vi "Init.vi"(8 "error in":errorcluster, 11 "CFG Base in":refnum<class "Red-y Pressure Control CFG.lvclass">) -> (0 "error out":errorcluster, 3 "CFG Base out":refnum<class "Red-y Pressure Control CFG.lvclass">)   [LabVIEW 2024, in "Red-y Pressure Control CFG.lvclass"]
uses:
  Red-y Pressure Control CFG.lvclass
  Red-y Pressure Control CFG.lvclass/Red-y Pressure Control CFG.ctl
  Configurations/CFG Base/CFG Base.lvclass/CFG Base.ctl
  f61d1269-8a73-4422-950f-b7b3d93ad04d.vi
  3e784602-24e4-4a87-8e8a-87b1468842a3.vi
  f61d1269-8a73-4422-950f-b7b3d93ad04d.vi/a4169a97-72fc-4003-a778-603cf20cafa0.vi
  3e784602-24e4-4a87-8e8a-87b1468842a3.vi/a4169a97-72fc-4003-a778-603cf20cafa0.vi
  <vilib>/JDP Science/JSONtext/Find Item.vi
  <vilib>/JDP Science/JSONtext/Next JSON Value.vi
  <vilib>/JDP Science/JSONtext/String Subset.vi
  <vilib>/JDP Science/JSONtext/Parsing/Advance past next JSON Value (inlined COPY).vi
  <vilib>/JDP Science/JSONtext/Parsing/Advance past whitespace.vi
  <vilib>/JDP Science/JSONtext/Parsing/Advance past String.vi
  <vilib>/JDP Science/JSONtext/Parsing/Advance past Number.vi
  <vilib>/JDP Science/JSONtext/Parsing/Advance past Line Ending.vi
  <vilib>/JDP Science/JSONtext/Parsing/Parse Full Path or Item Name.vi
  <vilib>/JDP Science/JSONtext/Parsing/Advance past Array.vi
  <vilib>/JDP Science/JSONtext/Parsing/Advance past Object.vi
  <vilib>/JDP Science/JSONtext/support/Error Cluster From Code.vi
  <vilib>/JDP Science/JSONtext/Offset/Find Item Locations by Path.vi
  <vilib>/JDP Science/JSONtext/JSON text to Variant.vi
  <vilib>/Utility/error.llb/Error Cluster From Error Code.vi
  <vilib>/JDP Science/JSONtext/LVClass Serializer/JSONtext LVClass Serializer.lvclass
  Voegtlin_NI_SMART_Modbus_Drivers/Voegtlin_NI_SMART_Modbus_Drivers.lvlib
  Configurations/CFG Base/CFG Base.lvclass
  Configurations/CFG JSON/CFG JSON.lvclass
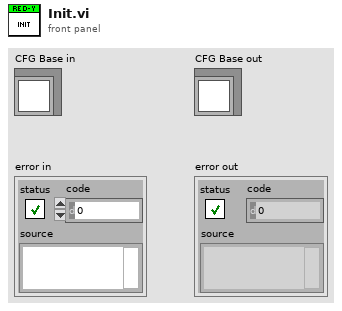
[diagram p1: front panel]
types:
  T1 = cluster{"COM Port Selected":string, "Data out":i32}
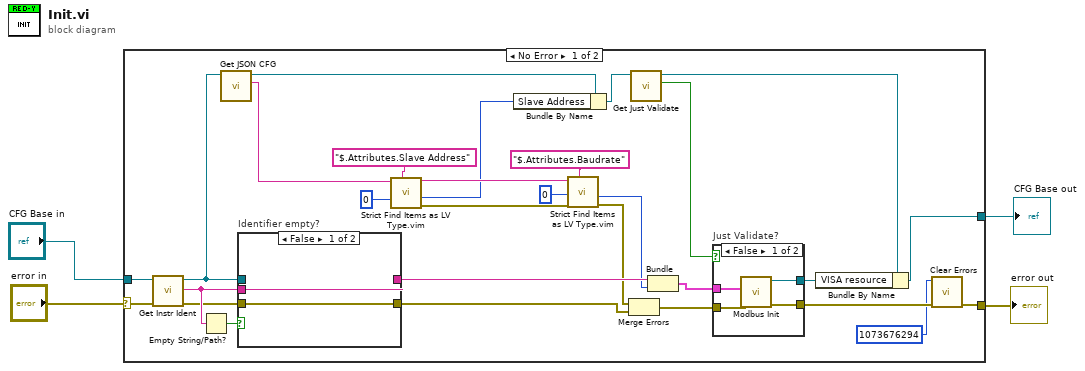
[diagram p0: block diagram]
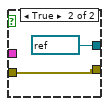
[diagram p2: hidden frame]
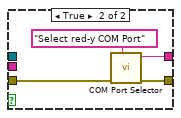
[diagram p3: hidden frame]
diagram:
  n1 = case shown="No Error" "error in" {
    selector: "error in" -> [w33 w46]
    tunnel: "CFG Base in" -> [w32 w47]
    tunnel: [w30 w47] -> w2
    tunnel: [w21 w46] -> w1
    frame No Error {
      n2 = call-dynamic "Get Instr Ident.vi"("error in"=w33, "CFG JSON in"=w32) -> ("error out"=w24:errorcluster, "Instr Ident"=w29:string, "CFG JSON out"=w25:refnum<class "Red-y Pressure Control CFG.lvclass">)  [unwired: 7 in]
      n3 = Empty String/Path?(string/path=w29) -> (empty?=w31:bool)
      n4 = call "Get JSON CFG.vi"("CFG JSON in"=w25) -> ("<JSON> CFG"=w9:string, "CFG JSON out"=w7:refnum<class "Red-y Pressure Control CFG.lvclass">)  [unwired: 9 in]
      n5 = case "Identifier empty?" shown="False" w31 {
        tunnel: w24 -> [w40 w42]
        tunnel: w29 -> [w41 _]
        tunnel: [w40 w45] -> w16
        tunnel: [w41 w43] -> w26
        tunnel: w25 -> [_ _]
        frame False {
        }
        frame True {
          n6 = call "COM Port Selector.vi"("Title"="Select red-y COM Port", "error in"=w42) -> ("error out"=w45:errorcluster, "COM Port Selected"=w43:string)  [unwired: 7 in]
        }
      }
      n7 = call "Strict Find Items as LV Type.vim"("$Path or Item Name"="$.Attributes.Slave Address", "Data Type and Default Value"=0, "<JSON>"=w9) -> ("error out"=w10:errorcluster, "Data out"=w5:i32, "<JSON> duplicate"=w11:string)  [unwired: 6 in]
      n8 = Bundle By Name(cluster=w7, "Slave Address"=w5) -> (w6:refnum<class "Red-y Pressure Control CFG.lvclass">)
      n9 = call "Strict Find Items as LV Type.vim"("$Path or Item Name"="$.Attributes.Baudrate", "error in"=w10, "Data Type and Default Value"=0, "<JSON>"=w11) -> ("error out"=w15:errorcluster, "Data out"=w13:i32)  [unwired: 5 in, 1 out]
      n10 = Merge Errors(w15, w16) -> (w23:errorcluster)
      n11 = call "Get Just Validate.vi"("CFG Base in"=w6) -> ("Just Validate"=w18:bool, "CFG Base out"=w19:refnum<class "Red-y Pressure Control CFG.lvclass">)  [unwired: 9 in]
      n12 = Bundle("COM Port Selected"=w26, "Data out"=w13) -> (w22:T1)  [unwired: 1 in]
      n13 = case "Just Validate?" shown="False" w18 {
        tunnel: [w37 refnum<visa-resource-name> "SIM" ("VISA resource out")] -> w28
        tunnel: [w36 w39] -> w27
        tunnel: w23 -> [w35 w39]
        tunnel: w22 -> [w34 _]
        frame False {
          n14 = call "Modbus Init.vi"("error in (no error)"=w35, "Modbus Port (Port, Baudrate)"=w34) -> ("error out"=w36:errorcluster, "VISA resource out"=w37:refnum<visa-resource-name>)  [unwired: 8 in]
        }
        frame True {
        }
      }
      n15 = Bundle By Name(cluster=w19, "VISA resource"=w28) -> (w30:refnum<class "Red-y Pressure Control CFG.lvclass">)
      n16 = call <vilib>:"Clear Errors.vi"("error in (no error)"=w27, "specific error code to clear (0: all)"=1073676294) -> ("error out"=w21:errorcluster)  [unwired: 4 in, 1 out]
    }
    frame Error {
    }
  }
  "error out" <- w1
  "CFG Base out" <- w2
